vi "libssh2_agent_publickey_refnum_get.vi"(8 "error in (no error)":errorcluster, 11 "public key":T1) -> (0 "error out":errorcluster, 2 "libssh2_agent_publickey*":u64)   [LabVIEW 2013, in "libssh2.lvlib"]
doc: "Gets the pointer to libssh2_agent_publickey associated with <B>public key</B>."
uses:
  libssh2.lvlib
  libssh2_agent_publickey_refnum.ctl
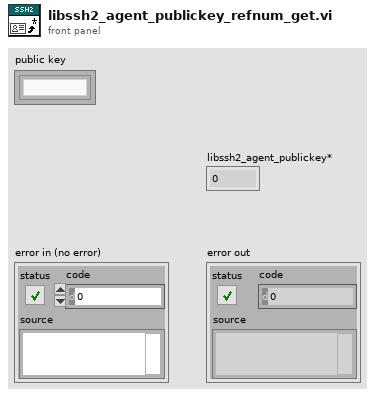
[diagram p1: front panel]
types:
  T1 = typedef "libssh2.lvlib/libssh2_agent_publickey_refnum.ctl" = refnum<k1>
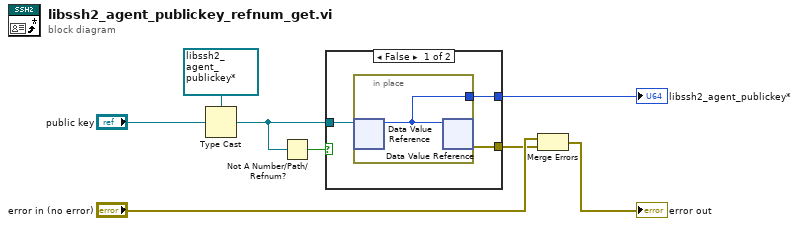
[diagram p0: block diagram]
diagram:
  n1 = Type Cast(type=refnum<data-value> refnum ("data value reference"), x="public key") -> (*(type *) &x=w2:refnum<data-value>)
  n2 = Not A Number/Path/Refnum?(number/path/refnum=w2) -> (NaN/Path/Refnum?=w1:bool)
  n3 = case shown="False" w1 {
    tunnel: w2 -> [w11 _]
    tunnel: [w10 _] -> w7
    tunnel: [w9 _] -> w3
    frame False {
      n4 = in-place {
        in-place-border: [w12] -> w10
        n5 = in-place-dvr #1(w11) -> (w12:u64)  [unwired: 1 out]
        n6 = in-place-dvr #1(w12) -> (w9:errorcluster)  [unwired: 1 out]
      }
    }
    frame True {
    }
  }
  "libssh2_agent_publickey*" <- w7
  n7 = Merge Errors("error in (no error)", w3) -> (→"error out":errorcluster)
